vi "Destroy.vi"(6 "Sender":refnum<class "Sender.lvclass">, 11 "Destroy in":refnum<class "Destroy.lvclass">) -> (0 "Error out":errorcluster, 3 "Destroy out":refnum<class "Destroy.lvclass">)   [LabVIEW 2025, in "jettl.lvlib" / "Destroy Msg.lvlib" / "Destroy.lvclass"]
uses:
  Destroy.lvclass
  Sender/Sender/Sender.lvclass
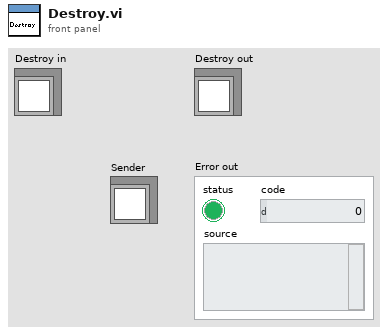
[diagram p1: front panel]
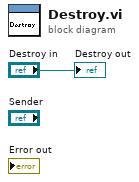
[diagram p0: block diagram]
diagram:
  "Destroy out" <- "Destroy in"
